vi "ValidateInputs.vi"(8 "error in":errorcluster, 9 "Supported Devices":u32[](array[numeric]), 10 "TargetInfoHistory":T1 {"IPTargetList"."Target RT Info List"."ProdID" format="%.0x"; "USBTargetList"."Target RT Info List"."ProdID" format="%.0x"; "WiFiTargetList"."Target RT Info List"."ProdID" format="%.0x"; "GenericTargetList"."Target RT Info List"."ProdID" format="%.0x"}, 11 "UI Ref Cluster":T4) -> (0 "error out":errorcluster, 2 "Error Message Array":string[](array[string]), 3 "UI Ref Cluster Out":T4)   [LabVIEW 2021, in "myRIOMetaDataObj.lvclass"]
uses:
  myRIOMetaDataObj.lvclass
  WizardUIRef.ctl
  AvailableTargets.ctl
  TargetInfoHistory.ctl
  TargetListInfo.ctl
  <resource>/myRIO/Target Info.ctl
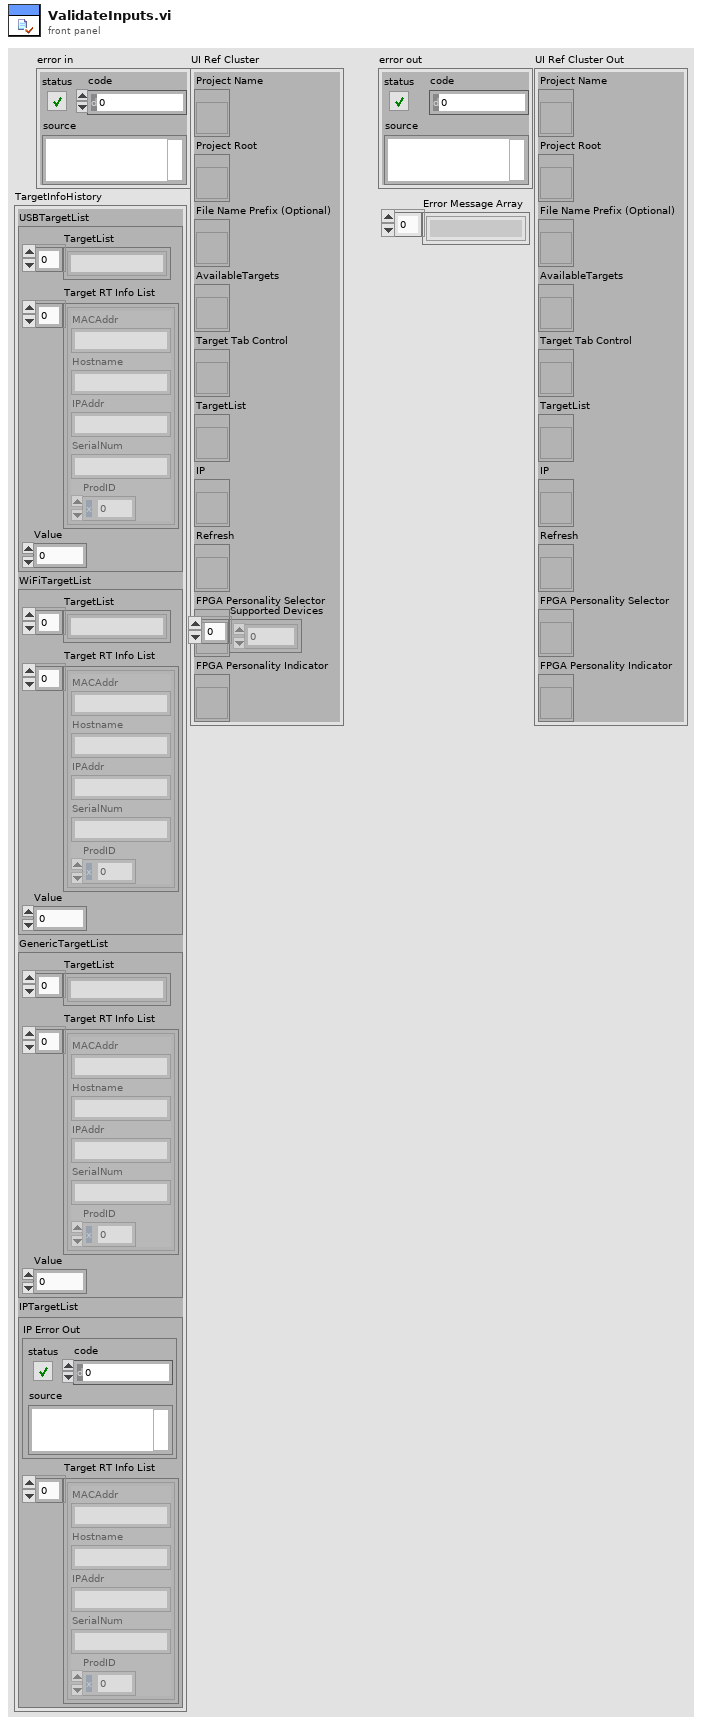
[diagram p1: front panel]
types:
  T1 = typedef "myRIOMetaDataObj.lvclass/TargetInfoHistory.ctl" = cluster{"USBTargetList":T2, "WiFiTargetList":T2, "GenericTargetList":T2, "IPTargetList":cluster{"IP Error Out":errorcluster, "Target RT Info List":T3[]}}
  T2 = typedef "myRIOMetaDataObj.lvclass/TargetListInfo.ctl" = cluster{"TargetList":string[], "Value":i32, "Target RT Info List":T3[]}
  T3 = typedef "Target Info.ctl" = cluster{"MACAddr":string, "Hostname":string, "IPAddr":string, "SerialNum":string, "ProdID":u32}
  T4 = typedef "myRIOMetaDataObj.lvclass/WizardUIRef.ctl" = cluster{"Project Name":refnum<vi>, "Project Root":refnum<vi>, "File Name Prefix (Optional)":refnum<vi>, "AvailableTargets":refnum<vi>, "Target Tab Control":refnum<vi>, "TargetList":refnum<vi>, "IP":refnum<vi>, "Refresh":refnum<vi>, "FPGA Personality Selector":refnum<vi>, "FPGA Personality Indicator":refnum<vi>}
  T5 = typedef "myRIOMetaDataObj.lvclass/AvailableTargets.ctl" = enum32{"USBTarget", "WifiTarget", "NoSpecificTarget", "TargetIP"}
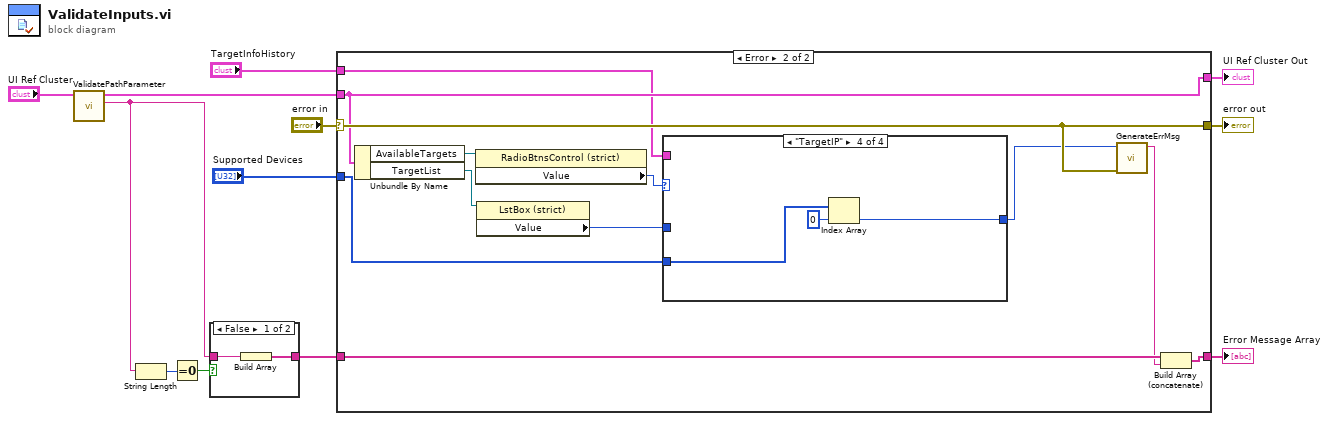
[diagram p0: block diagram]
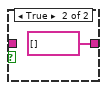
[diagram p2: hidden frame]
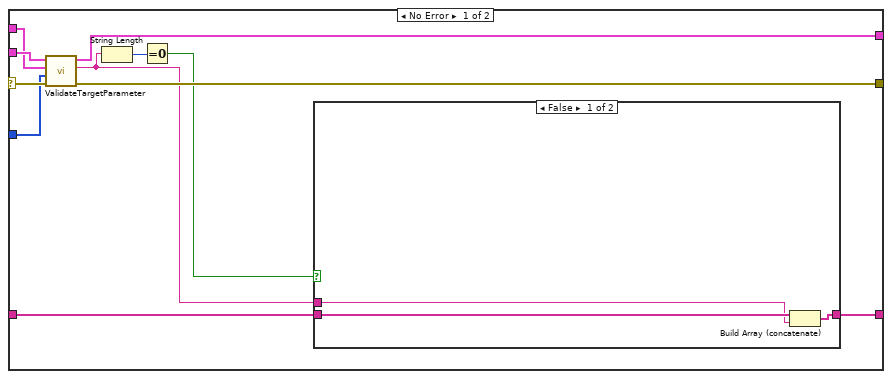
[diagram p3: hidden frame]
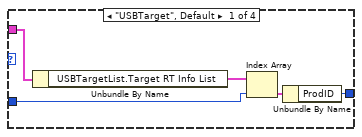
[diagram p5: hidden frame]
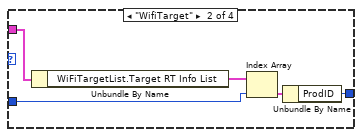
[diagram p6: hidden frame]
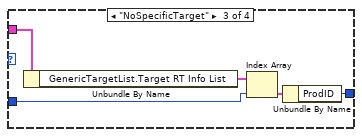
[diagram p7: hidden frame]
diagram:
  n1 = call "ValidatePathParameter.vi"("UI Ref Cluster"="UI Ref Cluster") -> ("Error Message"=w5:string, "UI Ref Cluster Out"=w9:T4)  [unwired: 8 in, 1 out]
  n2 = String Length(string=w5) -> (length=w7:i32)
  n3 = Equal To 0?(x=w7) -> (x = 0?=w6:bool)
  n4 = case shown="False" w6 {
    tunnel: [w14 string[] []] -> w4
    tunnel: w5 -> [w13 _]
    frame False {
      n5 = Build Array(w13) -> (w14:string[])
    }
    frame True {
    }
  }
  n6 = case shown="Error" "error in" {
    selector: "error in" -> [w19 w40]
    tunnel: [w25 w40] -> w11
    tunnel: w9 -> [w20 w38]
    tunnel: [w24 w41] -> w3
    tunnel: [w26 w38] -> w10
    tunnel: w4 -> [w18 w42]
    tunnel: "TargetInfoHistory" -> [w17 w33]
    tunnel: "Supported Devices" -> [w16 w31]
    frame No Error {
      n7 = call "ValidateTargetParameter.vi"("error in"=w19, "Supported Devices"=w16, "TargetInfoHistory"=w17, "UI Ref Cluster"=w20) -> ("error out"=w25:errorcluster, "Error Message"=w23:string, "UI Ref Cluster Out"=w26:T4)  [unwired: 5 in]
      n8 = String Length(string=w23) -> (length=w22:i32)
      n9 = Equal To 0?(x=w22) -> (x = 0?=w21:bool)
      n10 = case shown="False" w21 {
        tunnel: w18 -> [w29 w30]
        tunnel: [w27 w30] -> w24
        tunnel: w23 -> [w28 _]
        frame False {
          n11 = Build Array (concatenate)(w29, w28) -> (w27:string[])
        }
        frame True {
        }
      }
    }
    frame Error {
      n12 = Unbundle By Name(w38) -> ("AvailableTargets"=w37:refnum<vi>, "TargetList"=w35:refnum<vi>)
      n13 = property class="RadioBtnsControl (strict)"(reference=w37) -> ("Value"=w36:T5)  [unwired: 1 in, 2 out]
      n14 = property class="LstBox (strict)"(reference=w35) -> ("Value"=w34:i32)  [unwired: 1 in, 2 out]
      n15 = case shown="\"TargetIP\"" w36 {
        tunnel: w34 -> [w45 w50 w55 _]
        tunnel: w33 -> [w47 w52 w57 _]
        tunnel: [w43 w48 w53 w58] -> w32
        tunnel: w31 -> [_ _ _ w60]
        frame "USBTarget", Default {
          n16 = Unbundle By Name(w47) -> ("USBTargetList.Target RT Info List"=w46:T3[])
          n17 = Index Array(array=w46, index=w45) -> (element=w44:T3)
          n18 = Unbundle By Name(w44) -> ("ProdID"=w43:u32)
        }
        frame "WifiTarget" {
          n19 = Unbundle By Name(w52) -> ("WiFiTargetList.Target RT Info List"=w51:T3[])
          n20 = Index Array(array=w51, index=w50) -> (element=w49:T3)
          n21 = Unbundle By Name(w49) -> ("ProdID"=w48:u32)
        }
        frame "NoSpecificTarget" {
          n22 = Unbundle By Name(w57) -> ("GenericTargetList.Target RT Info List"=w56:T3[])
          n23 = Index Array(array=w56, index=w55) -> (element=w54:T3)
          n24 = Unbundle By Name(w54) -> ("ProdID"=w53:u32)
        }
        frame "TargetIP" {
          n25 = Index Array(array=w60, index=0) -> (element=w58:u32)
        }
      }
      n26 = call "GenerateErrMsg.vi"("error in (no error)"=w40, "Device Model"=w32) -> ("Error Message"=w39:string)  [unwired: 8 in, 1 out]
      n27 = Build Array (concatenate)(w42, w39) -> (w41:string[])
    }
  }
  "error out" <- w11
  "Error Message Array" <- w3
  "UI Ref Cluster Out" <- w10
